vi "camera_acq_H_shutter_sub.vi"(7 "Exposure time (ms)":dbl, 8 "error in (no error)":errorcluster, 9 "Binning":dbl=1.0 format="%#_13g", 10 "Camera in":u32) -> (0 "error out":errorcluster, 1 "Image":u16[][](graph), 2 "Camera out":u32)   [LabVIEW 2018]
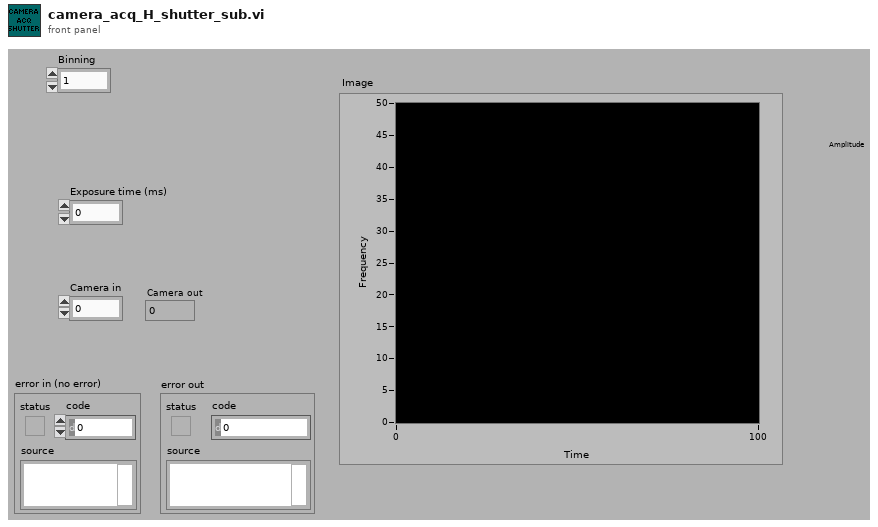
[diagram p1: front panel]
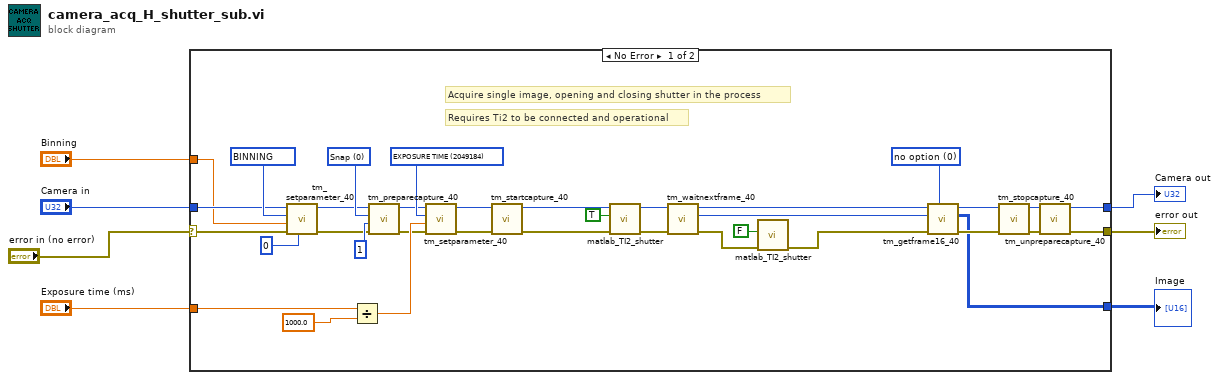
[diagram p0: block diagram]
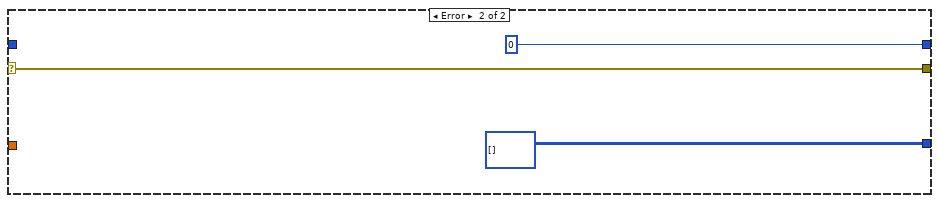
[diagram p2: hidden frame]
diagram:
  n1 = case shown="No Error" "error in (no error)" {
    selector: "error in (no error)" -> [w22 w44]
    tunnel: "Exposure time (ms)" -> [w31 _]
    tunnel: [w25 u32 0 ("Handle out")] -> w6
    tunnel: [w36 w44] -> w7
    tunnel: "Camera in" -> [w21 _]
    tunnel: [w32 u16[][] [] ("Data")] -> w2
    tunnel: "Binning" -> [w14 _]
    frame No Error {
      w19 = 0 items=["Snap", "Sequence"] ("Capture mode")
      w24 = u32 4215968 items=["SENSOR MODE"=4212128, "READOUT SPEED"=4211872, "READOUT DIRECTION"=4211904, "TRIGGER GLOBAL EXPOSURE"=2049680, "TRIGGER DELAY"=1066480, "INTERNAL TRIGGER HANDLING"=1066496, "SYNC READOUT SYSTEM BLANK"=1066528, "SENSOR TEMPERATURE"=2115232, "SENSOR COOLER STATUS"=2115280, "EXPOSURE TIME"=2049184, "DEFECT CORRECT MODE"=4670368, "BINNING"=4215968, "INTERNAL LINE SPEED"=4226000, "INTERNAL LINE INTERVAL"=4226016, "NUMBER OF OUTPUT TRIGGER CONNECTOR"=1852320, "OUTPUT TRIGGER SOURCE[0]"=1852576, "OUTPUT TRIGGER SOURCE[1]"=1852832, "OUTPUT TRIGGER SOURCE[2]"=1853088, "OUTPUT TRIGGER POLARITY[0]"=1852592, "OUTPUT TRIGGER POLARITY[1]"=1852848, "OUTPUT TRIGGER POLARITY[2]"=1853104, "OUTPUT TRIGGER ACTIVE[0]"=1852608, "OUTPUT TRIGGER ACTIVE[1]"=1852864, "OUTPUT TRIGGER ACTIVE[2]"=1853120, "OUTPUT TRIGGER DELAY[0]"=1852624, "OUTPUT TRIGGER DELAY[1]"=1852880, "OUTPUT TRIGGER DELAY[2]"=1853136, "OUTPUT TRIGGER PERIOD[0]"=1852640, "OUTPUT TRIGGER PERIOD[1]"=1852896, "OUTPUT TRIGGER PERIOD[2]"=1853152, "OUTPUT TRIGGER KIND[0]"=1852656, "OUTPUT TRIGGER KIND[1]"=1852912, "OUTPUT TRIGGER KIND[2]"=1853168, "OUTPUT TRIGGER BASE SENSOR[0]"=1852672, "OUTPUT TRIGGER BASE SENSOR[1]"=1852928, "OUTPUT TRIGGER BASE SENSOR[2]"=1853184, "OUTPUT TRIGGER PRE HSYNC COUNT"=1852704] ("Parameter")
      w29 = 0 items=["no option"=0, "high contrast"=16] ("Options")
      w41 = u32 2049184 items=["SENSOR MODE"=4212128, "READOUT SPEED"=4211872, "READOUT DIRECTION"=4211904, "TRIGGER GLOBAL EXPOSURE"=2049680, "TRIGGER DELAY"=1066480, "INTERNAL TRIGGER HANDLING"=1066496, "SYNC READOUT SYSTEM BLANK"=1066528, "SENSOR TEMPERATURE"=2115232, "SENSOR COOLER STATUS"=2115280, "EXPOSURE TIME"=2049184, "DEFECT CORRECT MODE"=4670368, "BINNING"=4215968, "INTERNAL LINE SPEED"=4226000, "INTERNAL LINE INTERVAL"=4226016, "NUMBER OF OUTPUT TRIGGER CONNECTOR"=1852320, "OUTPUT TRIGGER SOURCE[0]"=1852576, "OUTPUT TRIGGER SOURCE[1]"=1852832, "OUTPUT TRIGGER SOURCE[2]"=1853088, "OUTPUT TRIGGER POLARITY[0]"=1852592, "OUTPUT TRIGGER POLARITY[1]"=1852848, "OUTPUT TRIGGER POLARITY[2]"=1853104, "OUTPUT TRIGGER ACTIVE[0]"=1852608, "OUTPUT TRIGGER ACTIVE[1]"=1852864, "OUTPUT TRIGGER ACTIVE[2]"=1853120, "OUTPUT TRIGGER DELAY[0]"=1852624, "OUTPUT TRIGGER DELAY[1]"=1852880, "OUTPUT TRIGGER DELAY[2]"=1853136, "OUTPUT TRIGGER PERIOD[0]"=1852640, "OUTPUT TRIGGER PERIOD[1]"=1852896, "OUTPUT TRIGGER PERIOD[2]"=1853152, "OUTPUT TRIGGER KIND[0]"=1852656, "OUTPUT TRIGGER KIND[1]"=1852912, "OUTPUT TRIGGER KIND[2]"=1853168, "OUTPUT TRIGGER BASE SENSOR[0]"=1852672, "OUTPUT TRIGGER BASE SENSOR[1]"=1852928, "OUTPUT TRIGGER BASE SENSOR[2]"=1853184, "OUTPUT TRIGGER PRE HSYNC COUNT"=1852704] ("Parameter")
      # "Requires Ti2 to be connected and operational"
      # "Acquire single image, opening and closing shutter in the process"
      n2 = call <userlib>:"tm_setparameter_40.vi"("Index"=0, "error in (no error)"=w22, "Value in"=w14, "Parameter"=w24, "Handle in"=w21) -> ("error out"=w15:errorcluster, "Handle out"=w18:u32)  [unwired: 5 in]
      n3 = Divide(x=w31, y=1000.0) -> (x/y=w26:dbl)
      n4 = call <userlib>:"tm_preparecapture_40.vi"("error in (no error)"=w15, "Frames"=1, "Capture mode"=w19, "Handle in"=w18) -> ("error out"=w16:errorcluster, "Handle out"=w17:u32)  [unwired: 4 in, 2 out]
      n5 = call <userlib>:"tm_setparameter_40.vi"("error in (no error)"=w16, "Value in"=w26, "Parameter"=w41, "Handle in"=w17) -> ("error out"=w27:errorcluster, "Handle out"=w28:u32)  [unwired: 6 in]
      n6 = call <userlib>:"tm_startcapture_40.vi"("error in (no error)"=w27, "Handle in"=w28) -> ("error out"=w13:errorcluster, "Handle out"=w40:u32)  [unwired: 8 in]
      n7 = call "matlab_TI2_shutter.vi"("error in"=w13, "Shutter"=TRUE) -> ("error out"=w12:errorcluster)  [unwired: 9 in]
      n8 = call <userlib>:"tm_waitnextframe_40.vi"("error in (no error)"=w12, "Handle in"=w40) -> ("error out"=w11:errorcluster, "Frame Index"=w33:i32, "Handle out"=w39:u32)  [unwired: 6 in, 1 out]
      n9 = call "matlab_TI2_shutter.vi"("error in"=w11, "Shutter"=FALSE) -> ("error out"=w8:errorcluster)  [unwired: 9 in]
      n10 = call <userlib>:"tm_getframe16_40.vi"("Options"=w29, "error in (no error)"=w8, "Frame Index"=w33, "Handle in"=w39) -> ("error out"=w38:errorcluster, "Data"=w32:u16[][], "Handle out"=w34:u32)  [unwired: 4 in, 1 out]
      n11 = call <userlib>:"tm_stopcapture_40.vi"("error in (no error)"=w38, "Handle in"=w34) -> ("error out"=w37:errorcluster, "Handle out"=w35:u32)  [unwired: 8 in]
      n12 = call <userlib>:"tm_unpreparecapture_40.vi"("error in (no error)"=w37, "Handle in"=w35) -> ("error out"=w36:errorcluster, "Handle out"=w25:u32)  [unwired: 8 in]
    }
    frame Error {
    }
  }
  "Camera out" <- w6
  "error out" <- w7
  "Image" <- w2
